vi "Git_FindTagValue.vi"(8 "Error In":errorcluster, 10 "Tag Name":string="\\\"name\"", 11 "Text":string) -> (0 "Error Out":errorcluster, 2 "String Not Found?":bool, 3 "Value":string, 5 "Text after tag":string, 7 "Text before tag":string)   [LabVIEW 2012]
doc: "This VI will find the info for the corresponding tag from JSON styled text, and output the text before and after."
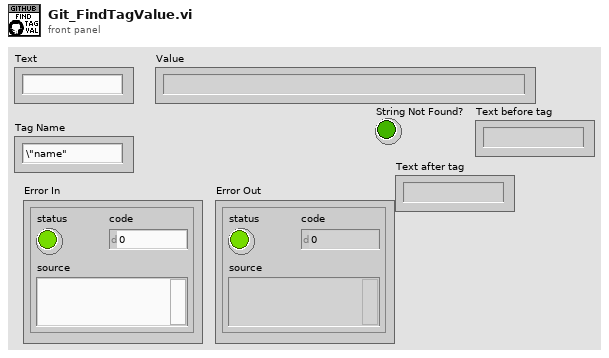
[diagram p1: front panel]
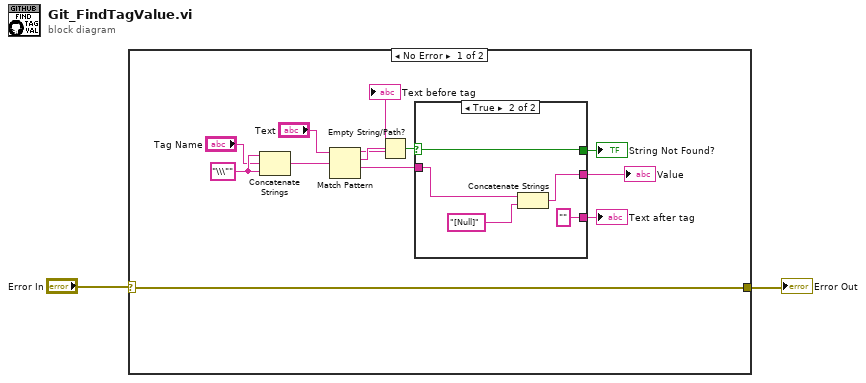
[diagram p0: block diagram]
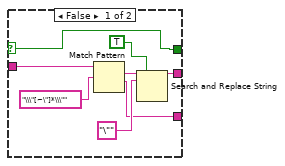
[diagram p2: hidden frame]
diagram:
  n1 = case shown="No Error" "Error In" {
    selector: "Error In" -> [w5 w28]
    tunnel: [w5 w28] -> w1
    frame No Error {
      w13 = "\\\"" ("string")
      n2 = Concatenate Strings(w13, "Tag Name", w13) -> (w14:string)
      n3 = Match Pattern(string="Text", regular expression=w14) -> (before substring=→"Text before tag":string, match substring=w8:string, after substring=w9:string)  [unwired: 1 in, 1 out]
      n4 = Empty String/Path?(string/path=w8) -> (empty?=w7:bool)
      n5 = case shown="True" w7 {
        selector: w7 -> [w16 w24]
        tunnel: [w22 w25] -> w10
        tunnel: w9 -> [w18 w27]
        tunnel: [w16 w24] -> w6
        tunnel: [w15 "" ("Text")] -> w3
        frame False {
          n6 = Match Pattern(string=w18, regular expression="\\\"[~\"]*\\\"") -> (match substring=w19:string, after substring=w15:string)  [unwired: 1 in, 2 out]
          n7 = Search and Replace String(replace all?=TRUE ("replace all? (F)"), input string=w19, search string="\"") -> (result string=w22:string)  [unwired: 5 in, 3 out]
        }
        frame True {
          n8 = Concatenate Strings(w27, "[Null]" ("result string")) -> (w25:string)
        }
      }
      "Value" <- w10
      "String Not Found?" <- w6
      "Text after tag" <- w3
    }
    frame Error {
    }
  }
  "Error Out" <- w1
